vi "Write Status.vi"(8 "error in (no error)":errorcluster, 10 "Weather Station Contents":T1, 11 "Weather Station in":refnum<class "Weather Station.lvclass">) -> (0 "error out":errorcluster, 3 "Weather Station out":refnum<class "Weather Station.lvclass">)   [LabVIEW 2018, in "Weather Station.lvclass"]
uses:
  Weather Station.lvclass
  Weather Station.lvclass/Weather Station.ctl
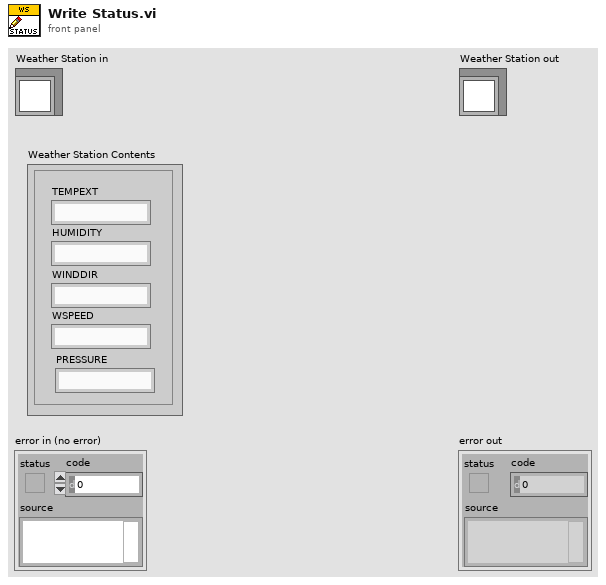
[diagram p1: front panel]
types:
  T1 = cluster{"TEMPEXT":string, "PRESSURE":string, "HUMIDITY":string, "WINDDIR":string, "WSPEED":string}
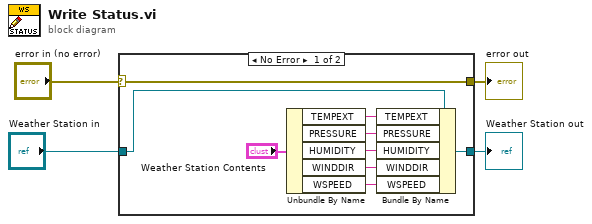
[diagram p0: block diagram]
diagram:
  n1 = case shown="No Error" "error in (no error)" {
    selector: "error in (no error)" -> [w13 w15]
    tunnel: [w13 w15] -> w3
    tunnel: [w11 w14] -> w1
    tunnel: "Weather Station in" -> [w12 w14]
    frame No Error {
      n2 = Unbundle By Name("Weather Station Contents") -> ("TEMPEXT"=w5:string, "PRESSURE"=w6:string, "HUMIDITY"=w7:string, "WINDDIR"=w8:string, "WSPEED"=w9:string)
      n3 = Bundle By Name(cluster=w12, "TEMPEXT"=w5, "PRESSURE"=w6, "HUMIDITY"=w7, "WINDDIR"=w8, "WSPEED"=w9) -> (w11:refnum<class "Weather Station.lvclass">)
    }
    frame Error {
    }
  }
  "error out" <- w3
  "Weather Station out" <- w1
